vi "Read Inbound URI.vi"(11 "Connection in":refnum<class "Connection.lvclass">) -> (2 "Inbound URI":string, 3 "Connection out":refnum<class "Connection.lvclass">)   [LabVIEW 2013, in "Connection_GOSPL.lvlib" / "Connection.lvclass"]
uses:
  Connection.lvclass
  Connection.lvclass/Connection.ctl
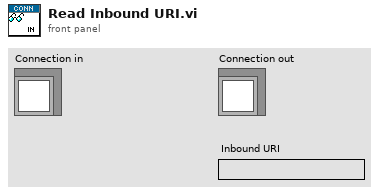
[diagram p1: front panel]
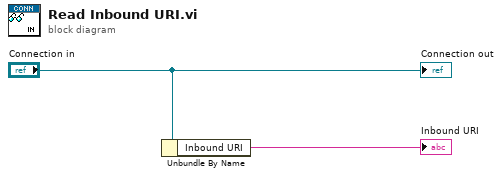
[diagram p0: block diagram]
diagram:
  n1 = Unbundle By Name("Connection in") -> ("Inbound URI"=→"Inbound URI":string)
  "Connection out" <- "Connection in"
